vi "mini_test_main_(QMH_ver).vi"() -> ()   [LabVIEW 2015]
doc: "This program is designed to work with CHROMA instruments, models 19052 and 19572, through the SERIAL RS232 or GPIB interfaces; whichever interface is chosen, it must be used in both.\nNOTE: This application was tested with the following interfaces: National Instruments GPIB-USB-HS and HS+, USB-A to RS-232 (DB9) Serial Adapter Cable Tripp Lite U209-000-R, 2 Port Industrial USB to Serial Adapter Hub ICUSB2322I. The one that gave the best result was the Startech interface.\n\nThe application takes configuration parameters from two files: config.ini and VISA_config.ini.\nThe first one configures the test mode and the delay time between the start of the second test and the start of the first one. And the second one configures communication parameters for the chosen interface.\n\nThe application has the ability to test in 4 different modes: The first two modes can perform Hi-Pot and GB testing simultaneously. The second two are single tests, one or the other, Hi-Pot or GB. The four possible modes are described as follows.\n\ntest_mode = 0, performs the sequence Hi-Pot then GB. The tests can be simultaneous or in sequence: Hi-Pot first and then GB. The start of the second one depends on the programmed delay time.\ntest_mode = 1, performs the sequence GB then Hi-Pot. The tests can be simultaneous or in sequence: GB first and then Hi-Pot. The start of the second test depends on the programmed delay time.\ntest_mode = 2, performs the Hi-Pot test only, and is the default test in case no mode is chosen in the config.ini configuration file.\ntest_mode = 3, performs the GB only GB test."
uses:
  controls/UI Data.ctl
  controls/HP Data.ctl
  controls/GB Data.ctl
  controls/Timer Data.ctl
  support/Message Queue/Enqueue Message (Array).vi
  support/Message Queue/Enqueue Message (Single).vi
  <vilib>/Utility/error.llb/Error Cluster From Error Code.vi
  <vilib>/ErrorRing/Error Ring.xnode
  support/Message Queue/Message Queue.lvlib
  support/User Event - Stop/User Event - Stop.lvlib
panel:
  in  "stp tmr":bool caption="stop"
  out "GB Pass/Fail":cluster{"PASS":bool, "FAIL":bool}
  out "HP Pass/Fail":cluster{"PASS":bool, "FAIL":bool}
  out "tst mod":T1(ring) caption="Test mode"
  out "tst time":dbl caption="total test time"
  out "overlap":dbl
  out "2d tst":dbl caption="test time 2"
  out "1st tst":dbl caption="test time 1"
  out "delay":dbl caption="delay time"
  out "GB test":dbl(slide) caption="GB test time [s]" scale=0.0..1.0 scale format="%#_3g"
  out "HP test":dbl(slide) caption="Hi-Pot test time [s]" scale=0.0..1.0 scale format="%#_3g"
  out "I/F type":string caption="Interface type"
  out "GB ID":string="\r\n" caption="GB Instrument ID"
  out "HP ID":string="\r\n" caption="Hi-Pot Instrument ID"
  out "GB tst reslts":string caption="GB test results"
  out "GB tst st":string caption="GB test status"
  out "HP tst rslts":string caption="Hi-Pot test results"
  out "HP tst st":string caption="Hi-Pot test status"
  out "Display":string
  in  "Stop test":bool
  in  "Start test":bool
  in  "Exit Button":bool
  # "QMH version"
  # "Hi-Pot test"
  # "GB test"
  # "Warning. This app is a proof of concept and has no other purpose, \nit is not intended for production. Use at your own risk."
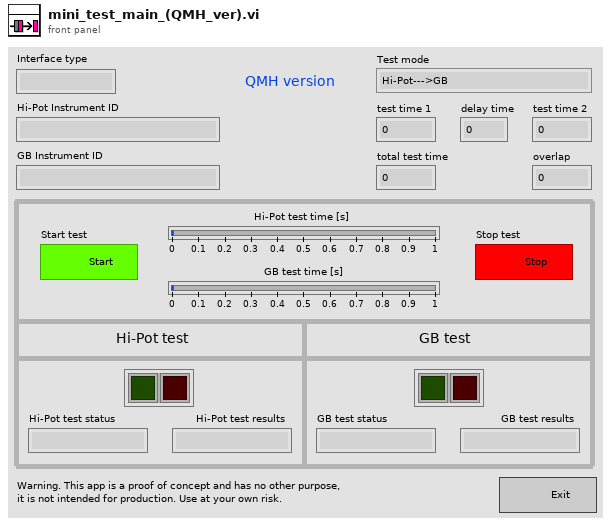
[diagram p1: front panel]
types:
  T1 = enum16{"Hi-Pot--->GB", "GB--->Hi-Pot", "Hi-Pot only", "GB only"}
  T2 = typedef "Timer Data.ctl" = cluster{"Delay time":dbl}
  T3 = typedef "GB Data.ctl" = cluster{"Status GB":string, "Results GB":string, "GB Pass/Fail":cluster{"PASS":bool, "FAIL":bool}}
  T4 = typedef "HP Data.ctl" = cluster{"Status HP":string, "Results HP":string, "HP Pass/Fail":cluster{"PASS":bool, "FAIL":bool}}
  T5 = typedef "UI Data.ctl" = cluster{"Delay Time":dbl, "prms":cluster{"1st tst":dbl, "2nd tst":dbl, "overlap":dbl, "tst time":dbl, "delay":dbl}, "test mode":enum16{"Hi-Pot--->GB", "GB--->Hi-Pot", "Hi-Pot only", "GB only"}, "Start Btn Refnum":refnum<vi>}
  T6 = cluster{"test mode number":string, "test mode":enum16{"Hi-Pot--->GB", "GB--->Hi-Pot", "Hi-Pot only", "GB only"}, "size":i32}
  T7 = cluster{"Rsrc name for 19572":refnum<visa-resource-name>, "Rsrc name for 19052":refnum<visa-resource-name>, "I/F type":string, "VISA2 Inst ID":string, "VISA1 Inst ID":string, "test mode":enum16{"Hi-Pot--->GB", "GB--->Hi-Pot", "Hi-Pot only", "GB only"}}
  T8 = typedef "Message Queue.lvlib/All Message Queues.ctl" = cluster{"Main":refnum<queue>, "GB Test":refnum<queue>, "HP Test":refnum<queue>, "Timer":refnum<queue>}
  T9 = enum8{"Enabled", "Disabled", "Disabled and Grayed Out"}
  T10 = cluster{"1st tst":dbl, "2nd tst":dbl, "overlap":dbl, "tst time":dbl, "delay":dbl}
  T11 = cluster{"1st test":dbl, "2nd test":dbl, "overlap":dbl, "test time":dbl, "delay":dbl}
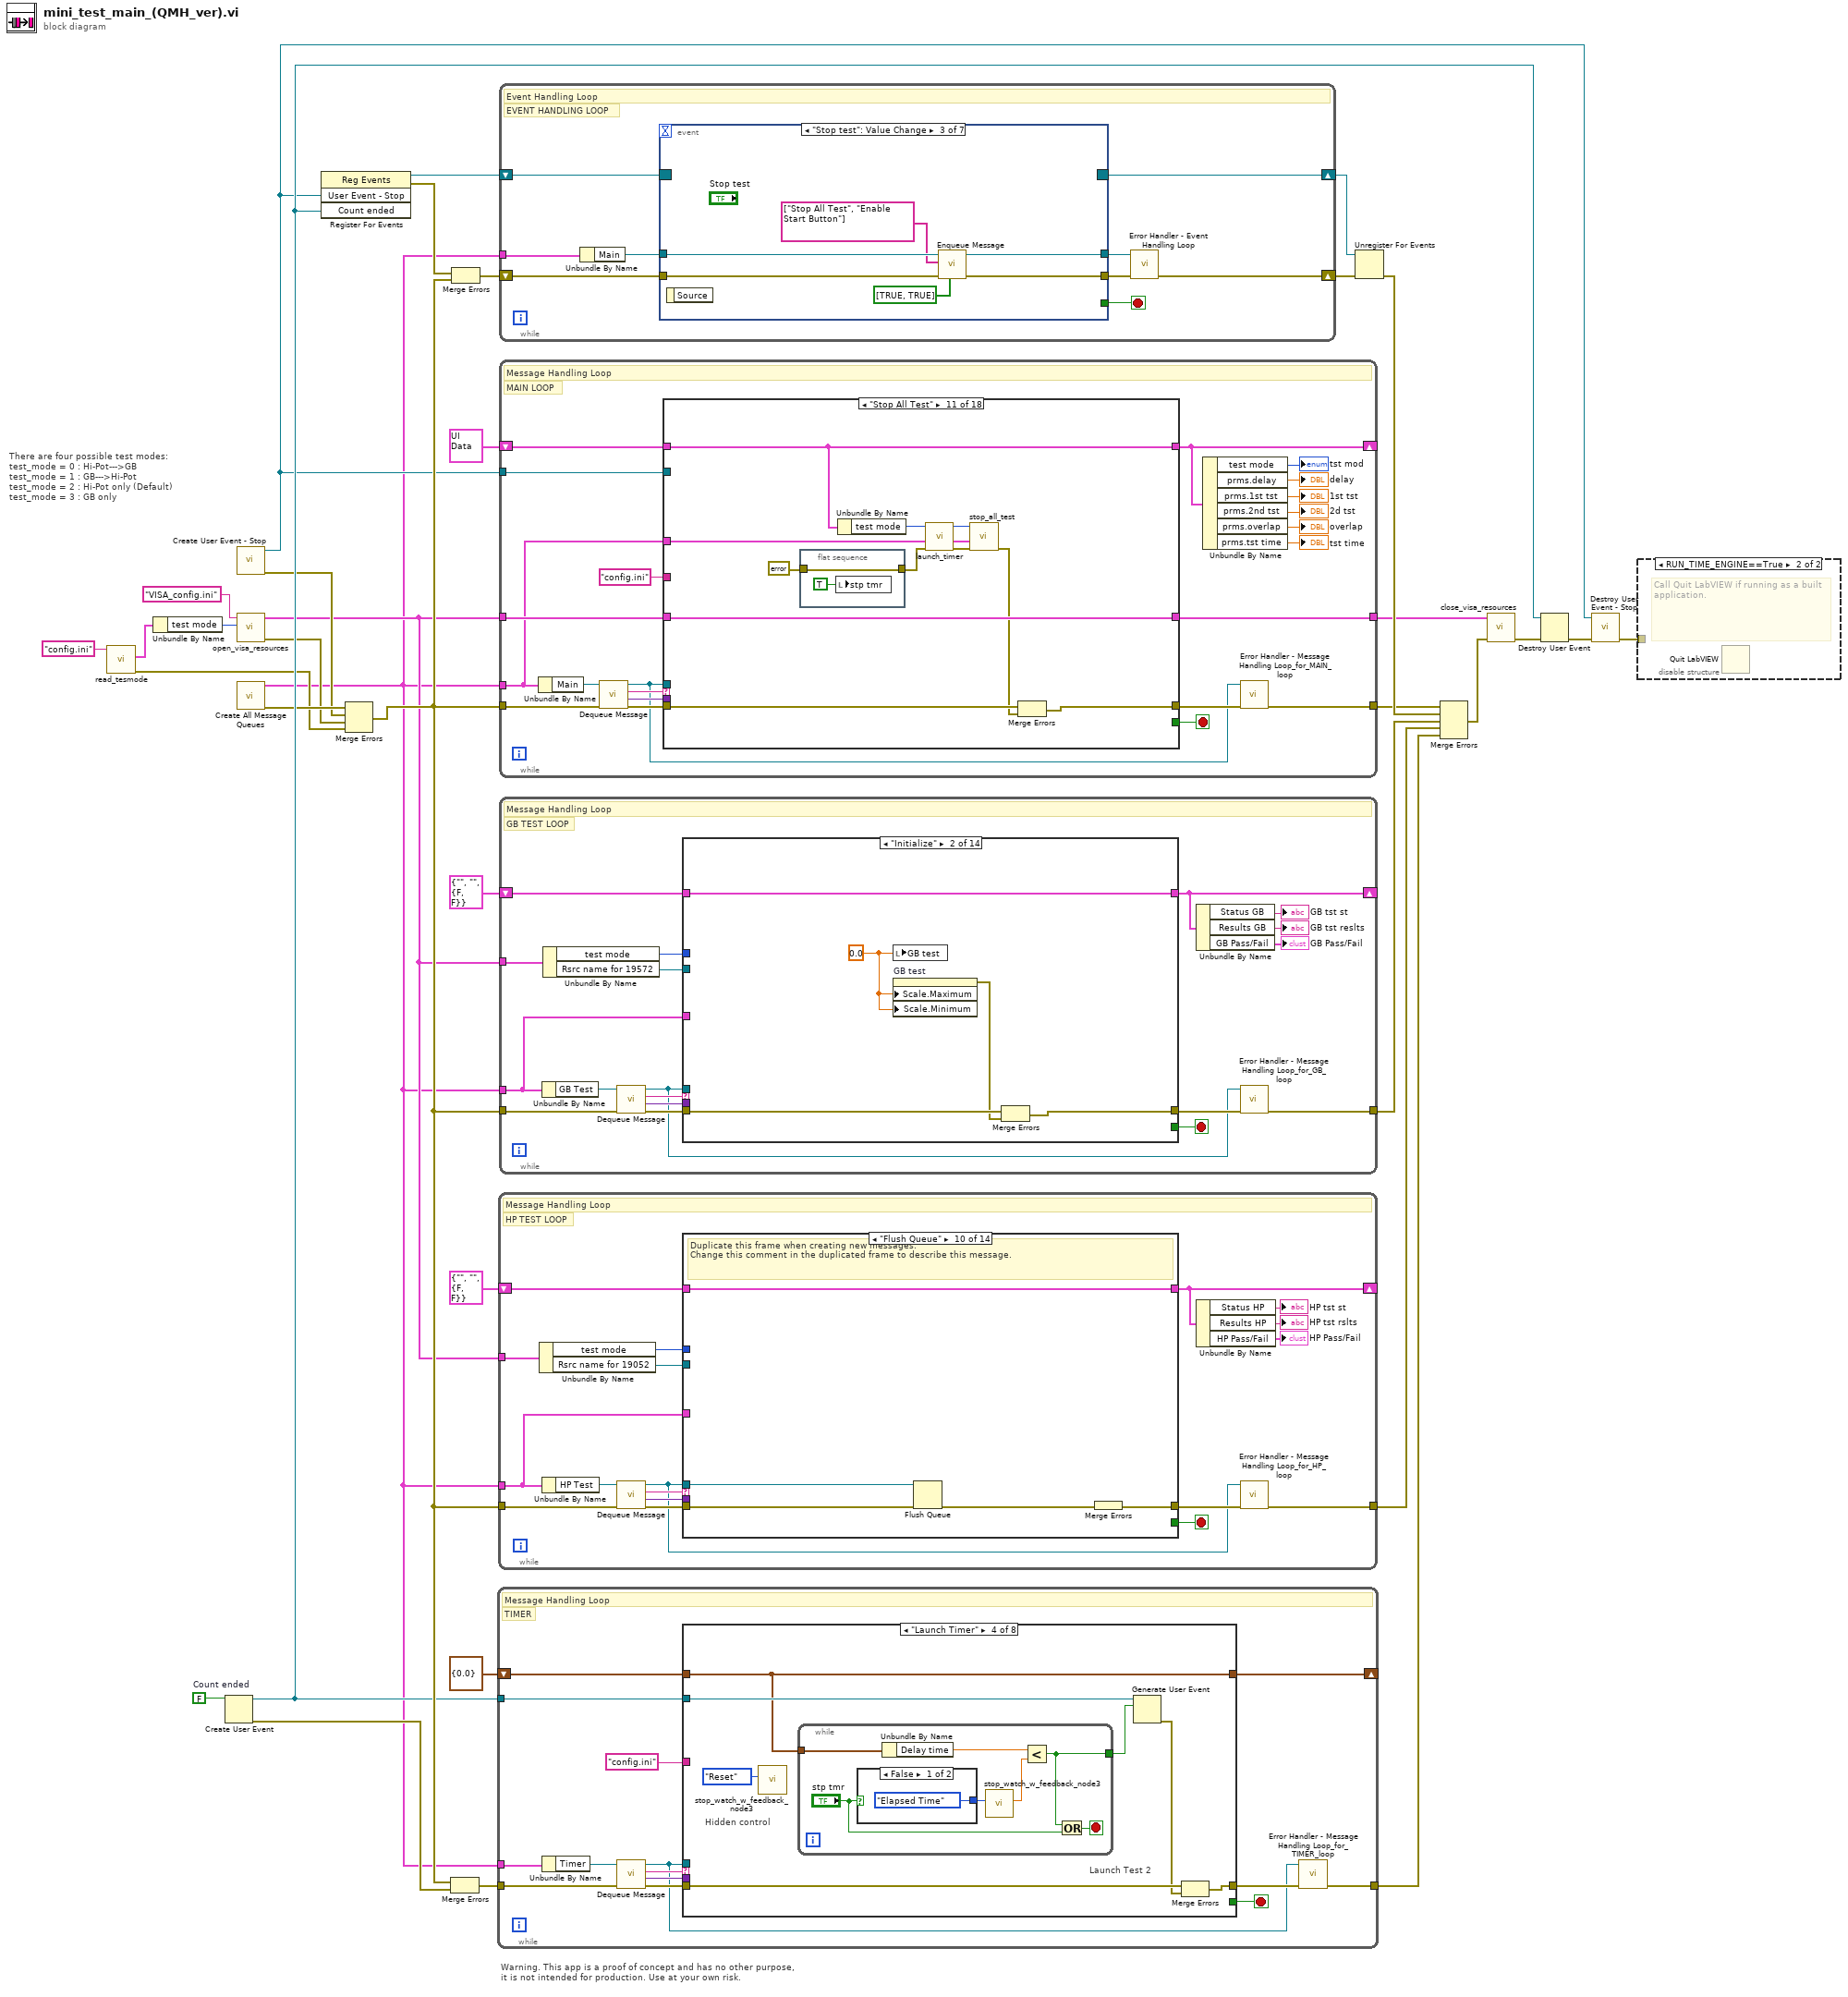
[diagram p0: block diagram]
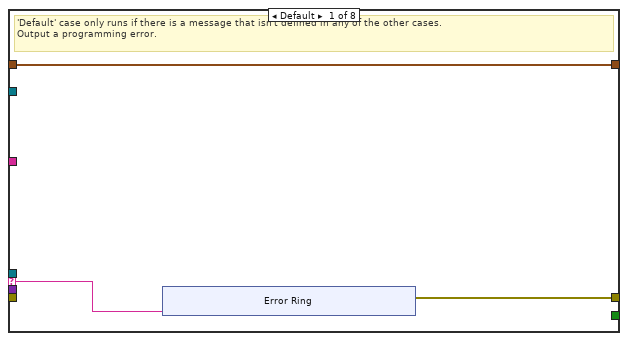
[diagram p2: hidden frame]
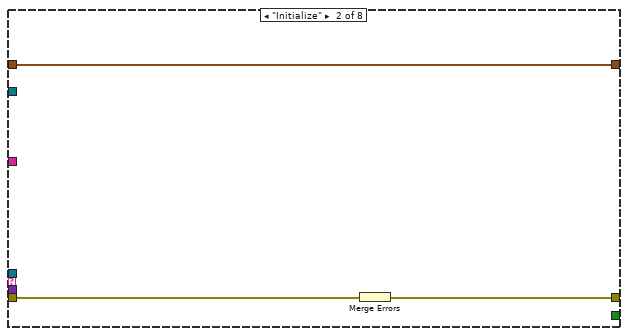
[diagram p3: hidden frame]
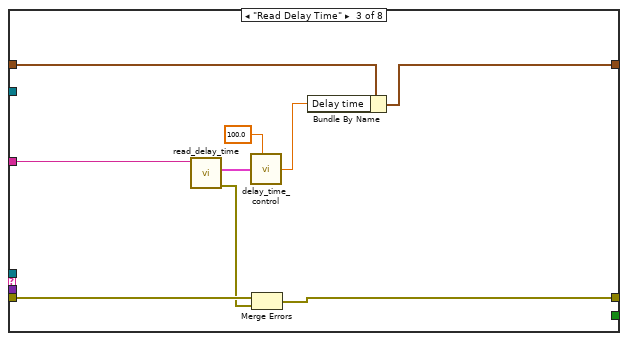
[diagram p4: hidden frame]
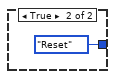
[diagram p5: hidden frame]
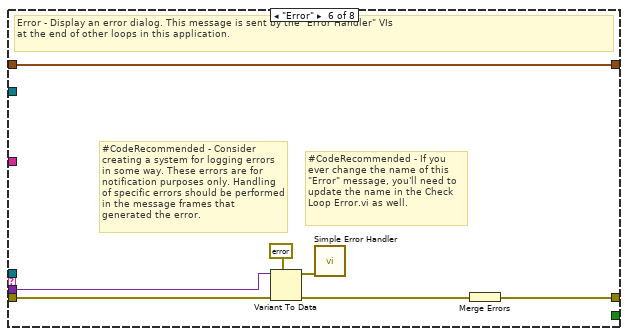
[diagram p7: hidden frame]
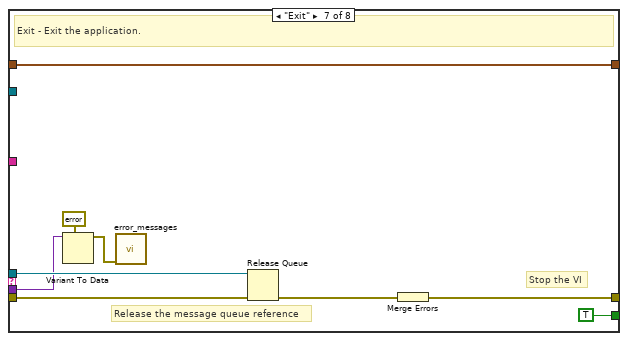
[diagram p8: hidden frame]
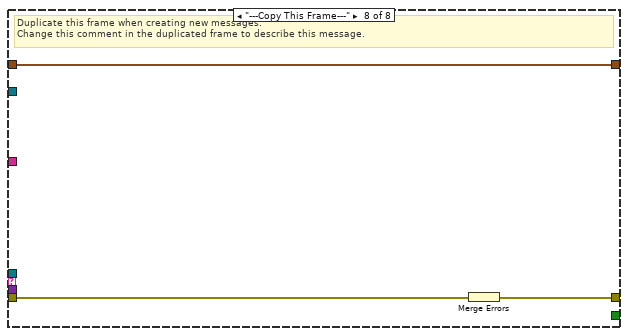
[diagram p9: hidden frame]
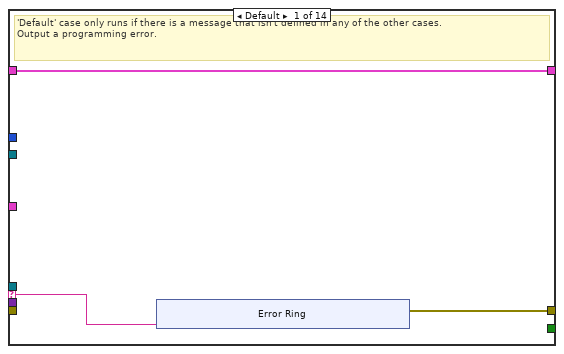
[diagram p10: hidden frame]
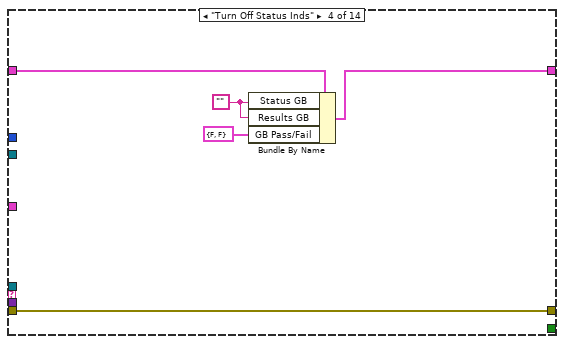
[diagram p12: hidden frame]
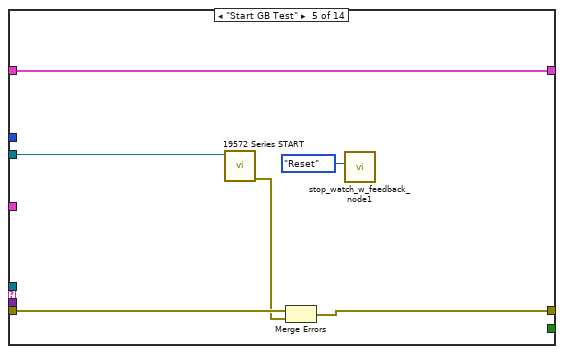
[diagram p13: hidden frame]
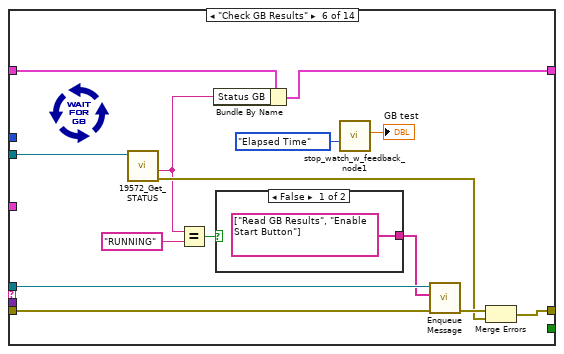
[diagram p14: hidden frame]
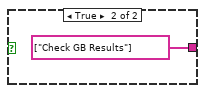
[diagram p15: hidden frame]
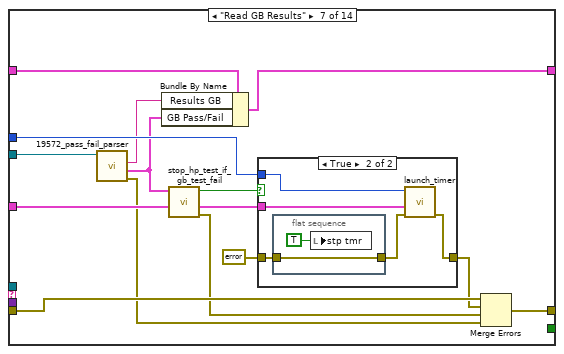
[diagram p16: hidden frame]
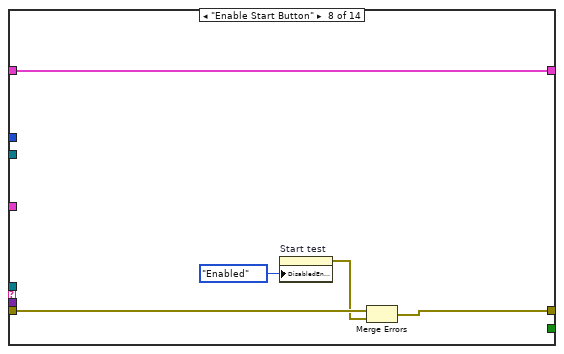
[diagram p18: hidden frame]
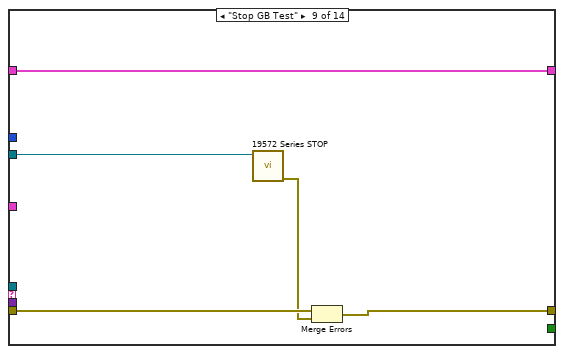
[diagram p19: hidden frame]
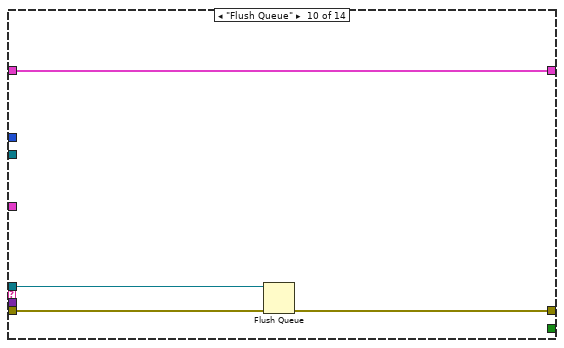
[diagram p20: hidden frame]
diagram:
  w13 = FALSE  # Count ended
  # "Warning. This app is a proof of concept and has no other purpose, \nit is not intended for production. Use at your own risk."
  # "There are four possible test modes:\ntest_mode = 0 : Hi-Pot--->GB\ntest_mode = 1 : GB--->Hi-Pot\ntest_mode = 2 : Hi-Pot only (Default)\ntest_mode = 3 : GB only"
  n1 = call "read_tesmode.vi"("config_file_name"="config.ini") -> ("error out"=w31:errorcluster, "test mode"=w17:T6)  [unwired: 8 in, 1 out]
  n2 = Unbundle By Name(w17) -> ("test mode"=w16:T1)
  n3 = Create User Event(user event datatype=w13) -> (user event=w34:refnum<user-event>, error out=w11:errorcluster)  [unwired: 1 in]
  n4 = call "Create User Event - Stop.vi"() -> ("error out"=w19:errorcluster, "User Event - Stop"=w29:refnum<user-event>)  [unwired: 10 in]
  n5 = call "open_visa_resources.vi"("test mode"=w16, "config file in"="VISA_config.ini") -> ("error out"=w32:errorcluster, "VISA out"=w6:T7)  [unwired: 8 in]
  n6 = call "Create All Message Queues.vi"() -> ("error out"=w33:errorcluster, "Message Queues out"=w5:T8)  [unwired: 10 in]
  n7 = register-events(w29, w34) -> (reference out=w25:refnum<event-registration>, error out=w30:errorcluster)  [unwired: 2 in]
  n8 = Merge Errors(w33, w19, w32, w31) -> (w35:errorcluster)
  n9 = Merge Errors(w35, w11) -> (w12:errorcluster)
  n10 = Merge Errors(w30, w35) -> (w4:errorcluster)
  n11 = while {
    shift-right: [w37] -> _
    shift-left: T2 {"Delay time"=0.0} ("Timer Data") -> [w49]
    tunnel: w12 -> [w48]
    tunnel: [w41] -> w7
    tunnel: w5 -> [w44]
    tunnel: w34 -> [w38]
    stop <- w45 stop-if-true
    # "TIMER"
    # "Message Handling Loop"
    n12 = Unbundle By Name(w44) -> ("Timer"=w43:refnum<queue>)
    n13 = call "Dequeue Message.vi"("error in (no error)"=w48, "Message Queue"=w43) -> ("error out"=w47:errorcluster, "Message Data"=w46:variant, "Message"=w40:string, "dup Message Queue"=w36:refnum<queue>)  [unwired: 6 in]
    n14 = case "Message Cases" shown="\"Launch Timer\"" w40 {
      selector: w40 -> [w50 _ _ _ _ _ _ _]
      tunnel: w36 -> [_ _ _ _ _ _ w105 _]
      tunnel: w47 -> [_ w61 w70 w76 w89 w96 w101 w108]
      tunnel: [w51 w60 w71 w78 w89 w90 w102 w106] -> w42
      tunnel: w49 -> [w52 w62 w69 w73 w88 w95 w97 w107]
      tunnel: [w52 w62 w65 w73 w88 w95 w97 w107] -> w37
      tunnel: [_ _ _ _ _ _ TRUE _] -> w45
      tunnel: w46 -> [_ _ _ _ _ w94 w99 _]
      tunnel: "config.ini" -> [_ _ w67 _ _ _ _ _]
      tunnel: w38 -> [_ _ _ w77 _ _ _ _]
      frame Default {
        # "'Default' case only runs if there is a message that isn't defined in any of the other cases. \nOutput a programming error."
        n15 = xnode "Error Ring"("parameter 0"=w50) -> ("error out"=w51:errorcluster)
      }
      frame "Initialize" {
        n16 = Merge Errors(w61) -> (w60:errorcluster)
      }
      frame "Read Delay Time" {
        n17 = call "read_delay_time.vi"("config_file_name"=w67) -> ("error out"=w64:errorcluster, "values"=w68:cluster{"delay_time":string})  [unwired: 8 in, 1 out]
        n18 = call "delay_time_control.vi"("Higher limit"=100.0, "values in"=w68) -> ("delay time"=w63:dbl)  [unwired: 5 in]
        n19 = Merge Errors(w70, w64) -> (w71:errorcluster)
        n20 = Bundle By Name(cluster=w69, "Delay time"=w63) -> (w65:T2)
      }
      frame "Launch Timer" {
        # "Launch Test 2"
        # "Hidden control"
        n21 = call "stop_watch_w_feedback_node3.vi"("Command"=enum16{"Elapsed Time", "Reset"}."Reset") -> ()  [unwired: 10 in, 1 out]
        n22 = while {
          tunnel: w73 -> [w85]
          tunnel: [w80] -> w72
          stop <- w84 stop-if-true
          n23 = case shown="False" "stp tmr" {
            tunnel: [enum16{"Elapsed Time", "Reset"}."Elapsed Time" ("Command") enum16{"Elapsed Time", "Reset"}."Reset" ("Command")] -> w83
            frame False {
            }
            frame True {
            }
          }
          n24 = Unbundle By Name(w85) -> ("Delay time"=w81:dbl)
          n25 = call "stop_watch_w_feedback_node3.vi"("Command"=w83) -> ("Elapsed Time"=w82:dbl)  [unwired: 10 in]
          n26 = Less?(x=w81, y=w82) -> (x < y?=w80:bool)
          n27 = Or(x=w80, y="stp tmr") -> (x .or. y?=w84:bool)
        }
        n28 = Generate User Event(user event=w77, event data cluster=w72) -> (error out=w75:errorcluster)  [unwired: 2 in, 1 out]
        n29 = Merge Errors(w76, w75) -> (w78:errorcluster)
      }
      frame "Idle" {
      }
      frame "Error" {
        # "#CodeRecommended - If you ever change the name of this \"Error\" message, you'll need to update the name in the Check Loop Error.vi as well."
        # "#CodeRecommended - Consider creating a system for logging errors in some way. These errors are for notification purposes only. Handling of specific errors should be performed in the message frames that generated the error."
        # "Error - Display an error dialog. This message is sent by the \"Error Handler\" VIs \nat the end of other loops in this application."
        n30 = Variant To Data(error in=w96, type=errorcluster {"status"=FALSE, "code"=0, "source"=""} ("error constant"), Variant=w94) -> (data=w92:errorcluster, error out=w91:errorcluster)
        n31 = call <vilib>:"Simple Error Handler.vi"("error in (no error)"=w92) -> ()  [unwired: 4 in, 5 out]
        n32 = Merge Errors(w91) -> (w90:errorcluster)
      }
      frame "Exit" {
        # "Stop the VI"
        # "Release the message queue reference"
        # "Exit - Exit the application."
        n33 = Variant To Data(type=errorcluster {"status"=FALSE, "code"=0, "source"=""} ("error constant"), Variant=w99) -> (data=w98:errorcluster)  [unwired: 1 in, 1 out]
        n34 = call "error_messages.vi"("error in (no error)"=w98) -> ()  [unwired: 10 in, 1 out]
        n35 = Release Queue(queue=w105, error in (no error)=w101) -> (error out=w103:errorcluster)  [unwired: 1 in, 2 out]
        n36 = Merge Errors(w103) -> (w102:errorcluster)
      }
      frame "---Copy This Frame---" {
        # "Duplicate this frame when creating new messages.\nChange this comment in the duplicated frame to describe this message."
        n37 = Merge Errors(w108) -> (w106:errorcluster)
      }
    }
    n38 = call "Error Handler - Message Handling Loop_for_TIMER_loop.vi"("error in (no error)"=w42, "Message Queue"=w36) -> ("dup error in"=w41:errorcluster)  [unwired: 8 in, 1 out]
  }
  n39 = while {
    shift-right: [w119] -> _
    shift-left: T4 {"Status HP"="", "Results HP"="", "HP Pass/Fail"={"PASS"=FALSE, "FAIL"=FALSE}} ("HP Data") -> [w126]
    tunnel: w35 -> [w125]
    tunnel: [w114] -> w24
    tunnel: w6 -> [w121]
    tunnel: w5 -> [w111]
    stop <- w122 stop-if-true
    # "HP TEST LOOP"
    # "Message Handling Loop"
    n40 = Unbundle By Name(w121) -> ("test mode"=w110:T1, "Rsrc name for 19052"=w120:refnum<visa-resource-name>)
    n41 = Unbundle By Name(w111) -> ("HP Test"=w116:refnum<queue>)
    n42 = call "Dequeue Message.vi"("error in (no error)"=w125, "Message Queue"=w116) -> ("error out"=w124:errorcluster, "Message Data"=w123:variant, "Message"=w113:string, "dup Message Queue"=w109:refnum<queue>)  [unwired: 6 in]
    n43 = case "Message Cases" shown="\"Flush Queue\"" w113 {
      selector: w113 -> [w127 _ _ _ _ _ _ _ _ _ _ _ _ _]
      tunnel: w109 -> [_ _ _ _ _ w165 _ _ _ w206 _ _ w235 _]
      tunnel: w124 -> [_ w139 w143 w148 w153 w167 w185 w198 w200 w205 w212 w221 w231 w238]
      tunnel: [w128 w138 w143 w148 w152 w168 w184 w195 w202 w207 w213 w215 w232 w236] -> w115
      tunnel: w126 -> [w129 w141 w142 w145 w149 w163 w182 w197 w203 w208 w214 w220 w226 w237]
      tunnel: [w129 w141 w142 w144 w149 w162 w181 w197 w203 w208 w214 w220 w225 w237] -> w119
      tunnel: [_ _ _ _ _ _ _ _ _ _ _ _ TRUE _] -> w122
      tunnel: w123 -> [_ _ _ _ _ _ _ _ _ _ w211 w219 w229 _]
      tunnel: w120 -> [_ _ _ _ w154 w164 w183 _ w201 _ _ _ _ _]
      tunnel: w111 -> [_ _ _ _ _ _ w178 _ _ _ _ _ _ _]
      tunnel: w110 -> [_ _ _ _ _ _ w176 _ _ _ _ _ _ _]
      frame Default {
        # "'Default' case only runs if there is a message that isn't defined in any of the other cases. \nOutput a programming error."
        n44 = xnode "Error Ring"("parameter 0"=w127) -> ("error out"=w128:errorcluster)
      }
      frame "Initialize" {
        w140 = 0.0
        n45 = local write "HP test"(w140) -> ()
        n46 = property on="HP test" class="Slide (strict)"("Scale.Maximum"=w140, "Scale.Minimum"=w140) -> (error out=w137:errorcluster)  [unwired: 2 in, 1 out]
        n47 = Merge Errors(w139, w137) -> (w138:errorcluster)
      }
      frame "Idle" {
      }
      frame "Turn Off Status Inds" {
        w146 = ""
        n48 = Bundle By Name(cluster=w145, "Status HP"=w146, "Results HP"=w146, "HP Pass/Fail"=cluster{"PASS":bool, "FAIL":bool} {"PASS"=FALSE, "FAIL"=FALSE} ("GB Pass/Fail")) -> (w144:T4)
      }
      frame "Start HP Test" {
        n49 = call "19052 Series START.vi"("VISA resource in"=w154) -> ("error out"=w151:errorcluster)  [unwired: 9 in, 1 out]
        n50 = Merge Errors(w153, w151) -> (w152:errorcluster)
        n51 = call "stop_watch_w_feedback_node2.vi"("Command"=enum16{"Elapsed Time", "Reset"}."Reset") -> ()  [unwired: 10 in, 1 out]
      }
      frame "Check HP Results" {
        n52 = call "19052_Get_STATUS.vi"("VISA resource in"=w164) -> ("error out"=w158:errorcluster, "Status"=w157:string)  [unwired: 8 in, 1 out]
        n53 = Equal?(x=w157, y="RUNNING") -> (x = y?=w160:bool)
        n54 = Bundle By Name(cluster=w163, "Status HP"=w157) -> (w162:T4)
        n55 = case shown="False" w160 {
          tunnel: [string[] ["Read HP Results", "Enable Start Button"] string[] ["Check HP Results"]] -> w159
          frame False {
          }
          frame True {
          }
        }
        n56 = call "stop_watch_w_feedback_node2.vi"("Command"=enum16{"Elapsed Time", "Reset"}."Elapsed Time") -> ("Elapsed Time"=→"HP test":dbl)  [unwired: 10 in]
        n57 = call-poly "Enqueue Message.vi"("error in (no error)"=w167, "Message Array"=w159, "Message Queue"=w165) -> ("error out"=w166:errorcluster)  [unwired: 7 in, 1 out]
        n58 = Merge Errors(w166, w158) -> (w168:errorcluster)
      }
      frame "Read HP Results" {
        n59 = call "19052_pass_fail_parser.vi"("VISA resource in"=w183) -> ("error out"=w177:errorcluster, "Pass/Fail"=w179:cluster{"PASS":bool, "FAIL":bool}, "Code Results"=w180:string)  [unwired: 7 in, 1 out]
        n60 = Bundle By Name(cluster=w182, "Results HP"=w180, "HP Pass/Fail"=w179) -> (w181:T4)
        n61 = call "stop_gb_test_if_hp_test_fail.vi"("Message Queues in"=w178, "Pass/Fail"=w179) -> ("error out"=w171:errorcluster, "Message Queues out"=w174:T8, "Fail?"=w173:bool)  [unwired: 7 in]
        n62 = case shown="True" w173 {
          tunnel: [w186 w190] -> w172
          tunnel: errorcluster {"status"=FALSE, "code"=0, "source"=""} ("error constant") -> [w186 w189]
          tunnel: w176 -> [_ w188]
          tunnel: w174 -> [_ w187]
          frame False {
          }
          frame True {
            n63 = flat-sequence {
              tunnel: w189 -> [w192]
              tunnel: [w192] -> w191
              frame #0 {
                n64 = local write "stp tmr"(TRUE ("stp tmr")) -> ()
              }
            }
            n65 = call "launch_timer.vi"("error in (no error)"=w191, "Message Queues in"=w187, "test mode in"=w188) -> ("error out"=w190:errorcluster)  [unwired: 6 in, 2 out]
          }
        }
        n66 = Merge Errors(w185, w177, w172, w171) -> (w184:errorcluster)
      }
      frame "Enable Start Button" {
        n67 = property on="Start test" class="Bool"("DisabledEnum"=T9."Enabled" ("Disabled")) -> (error out=w194:errorcluster)  [unwired: 2 in, 1 out]
        n68 = Merge Errors(w198, w194) -> (w195:errorcluster)
      }
      frame "Stop HP Test" {
        n69 = call "19052 Series STOP.vi"("VISA resource in"=w201) -> ("error out"=w199:errorcluster)  [unwired: 9 in, 1 out]
        n70 = Merge Errors(w200, w199) -> (w202:errorcluster)
      }
      frame "Flush Queue" {
        # "Duplicate this frame when creating new messages.\nChange this comment in the duplicated frame to describe this message."
        n71 = Flush Queue(queue=w206, error in (no error)=w205) -> (error out=w204:errorcluster)  [unwired: 2 out]
        n72 = Merge Errors(w204) -> (w207:errorcluster)
      }
      frame "Update HP Display" {
        # "#CodeRecommended - If you wish to decouple the Message Handling Loop from your user interface, consider creating User Events (like the \"Stop\" event in this VI) to message the Event Handling Loop whenever the user interface needs updating."
        # "Update Display - Convert the message data to a string to display in the Data Display indicator."
        n73 = Variant To Data(error in=w212, type="", Variant=w211) -> (error out=w209:errorcluster)  [unwired: 1 out]
        n74 = Merge Errors(w209) -> (w213:errorcluster)
      }
      frame "Error" {
        # "#CodeRecommended - If you ever change the name of this \"Error\" message, you'll need to update the name in the Check Loop Error.vi as well."
        # "#CodeRecommended - Consider creating a system for logging errors in some way. These errors are for notification purposes only. Handling of specific errors should be performed in the message frames that generated the error."
        # "Error - Display an error dialog. This message is sent by the \"Error Handler\" VIs \nat the end of other loops in this application."
        n75 = Variant To Data(error in=w221, type=errorcluster {"status"=FALSE, "code"=0, "source"=""} ("error constant"), Variant=w219) -> (data=w217:errorcluster, error out=w216:errorcluster)
        n76 = call <vilib>:"Simple Error Handler.vi"("error in (no error)"=w217) -> ()  [unwired: 4 in, 5 out]
        n77 = Merge Errors(w216) -> (w215:errorcluster)
      }
      frame "Exit" {
        w224 = ""
        w228 = 0.0 ("HP test")
        # "Stop the VI"
        # "Release the message queue reference"
        # "#CodeNeeded - Add any required cleanup code here. Note that if 'Exit' was called as a result of an error, an error dialog will be displayed. Add any custom error handling for an 'Exit' condition here as well."
        # "Exit - Exit the application."
        n78 = Variant To Data(type=errorcluster {"status"=FALSE, "code"=0, "source"=""} ("error constant"), Variant=w229) -> (data=w223:errorcluster)  [unwired: 1 in, 1 out]
        n79 = call "error_messages.vi"("error in (no error)"=w223) -> ()  [unwired: 10 in, 1 out]
        n80 = Release Queue(queue=w235, error in (no error)=w231) -> (error out=w233:errorcluster)  [unwired: 1 in, 2 out]
        n81 = property on="HP test" class="Slide (strict)"("Scale.Maximum"=w228, "Scale.Minimum"=w228) -> (error out=w227:errorcluster)  [unwired: 2 in, 1 out]
        n82 = local write "HP test"(w228) -> ()
        n83 = Merge Errors(w233, w227) -> (w232:errorcluster)
        n84 = Bundle By Name(cluster=w226, "Status HP"=w224, "Results HP"=w224, "HP Pass/Fail"=cluster{"PASS":bool, "FAIL":bool} {"PASS"=FALSE, "FAIL"=FALSE}) -> (w225:T4)
      }
      frame "---Copy This Frame---" {
        # "Duplicate this frame when creating new messages.\nChange this comment in the duplicated frame to describe this message."
        n85 = Merge Errors(w238) -> (w236:errorcluster)
      }
    }
    n86 = Unbundle By Name(w119) -> ("Status HP"=→"HP tst st":string, "Results HP"=→"HP tst rslts":string, "HP Pass/Fail"=→"HP Pass/Fail":cluster{"PASS":bool, "FAIL":bool})
    n87 = call "Error Handler - Message Handling Loop_for_HP_loop.vi"("error in (no error)"=w115, "Message Queue"=w109) -> ("dup error in"=w114:errorcluster)  [unwired: 8 in, 1 out]
  }
  n88 = while {
    shift-right: [w246] -> w27
    shift-left: w25 -> [w247]
    tunnel: w5 -> [w242]
    shift-right: [w239] -> w26
    shift-left: w4 -> [w240]
    stop <- w244 stop-if-true
    # "EVENT HANDLING LOOP"
    # "Event Handling Loop"
    n89 = Unbundle By Name(w242) -> ("Main"=w241:refnum<queue>)
    n90 = event shown="[2] \"Stop test\": Value Change" {
      selector: w247 -> [_ _ _ _ _ _ _]
      dyn-events: [_ _ _ _ _ _ _] -> w246
      timeout: _ -> [_ _ _ _ _ _ _]
      tunnel: [_ _ _ _ _ _ TRUE ("Discard?")] -> w244
      tunnel: w241 -> [w253 w258 w271 w278 w281 w287 w291]
      tunnel: [w249 w255 w268 w277 w280 w284 w288] -> w245
      tunnel: [w252 w257 w270 w276 w281 w286 w291] -> w243
      tunnel: w240 -> [w251 w256 w269 w275 w280 w285 w288]
      event "Start test": Value Change {
        n91 = event-data() -> ()  [unwired: 1 in, 1 out]
        n92 = call-poly "Enqueue Message.vi"("error in (no error)"=w251, "Message Array"=string[] ["Launch Test 1", "Idle"], "Message Queue"=w253) -> ("error out"=w250:errorcluster, "dup Message Queue"=w252:refnum<queue>)  [unwired: 7 in]
        n93 = Merge Errors(w250) -> (w249:errorcluster)
      }
      event User Event {
        n94 = event-data() -> ("Count ended"=w254:bool)  [unwired: 1 in]
        n95 = case shown="True" w254 {
          tunnel: w258 -> [w260 w265]
          tunnel: [w260 w264] -> w257
          tunnel: w256 -> [w259 w263]
          tunnel: [w259 w262] -> w255
          frame False {
          }
          frame True {
            n96 = call-poly "Enqueue Message.vi"("error in (no error)"=w263, "Message Array"=string[] ["Launch Test 2", "Idle"], "Message Queue"=w265) -> ("error out"=w262:errorcluster, "dup Message Queue"=w264:refnum<queue>)  [unwired: 7 in]
          }
        }
      }
      event "Stop test": Value Change {
        n97 = event-data() -> ()  [unwired: 1 in, 1 out]
        n98 = call-poly "Enqueue Message.vi"("Priority Message? Array"=bool[] [TRUE, TRUE], "error in (no error)"=w269, "Message Array"=string[] ["Stop All Test", "Enable Start Button"], "Message Queue"=w271) -> ("error out"=w268:errorcluster, "dup Message Queue"=w270:refnum<queue>)  [unwired: 6 in]
      }
      event Panel Close? {
        # "Send the 'Confirm Quit' message if the user closes the panel of the VI. Discard the event so the 'Confirm Quit' message has a chance to run."
        n99 = event-data() -> ()  [unwired: 1 in, 1 out]
        n100 = call-poly "Enqueue Message.vi"("Priority Message? (F)"=TRUE, "error in (no error)"=w275, "Message Data"="Are you sure?", "Message"="Confirm Quit", "Message Queue"=w278) -> ("error out"=w277:errorcluster, "dup Message Queue"=w276:refnum<queue>)  [unwired: 5 in]
        n101 = event-data("Discard?"=TRUE) -> ()  [unwired: 1 in, 1 out]
      }
      event Application Instance Close {
        # "#CodeRecommended - When a project closes, all VIs within that project are aborted and leave memory. However, any code placed in this event frame is guaranteed to run to completion, so add any cleanup code that absolutely must happen here."
        n102 = event-data() -> ()  [unwired: 1 in, 1 out]
      }
      event "Exit Button": Value Change {
        n103 = event-data() -> ()  [unwired: 1 in, 1 out]
        n104 = call-poly "Enqueue Message.vi"("Priority Message? Array"=bool[] [TRUE, TRUE, TRUE], "error in (no error)"=w285, "Message Array"=string[] ["Turn Off Indicators", "Exit", "Enable Start Button"], "Message Queue"=w287) -> ("error out"=w284:errorcluster, "dup Message Queue"=w286:refnum<queue>)  [unwired: 6 in]
      }
      event User Event {
        # "The Message Handling Loop processed an \"Exit\" message, which fired this event to stop the Event Handling Loop."
        n105 = event-data() -> ()  [unwired: 1 in, 1 out]
        n106 = local write "Display"("\"Exit\" button pressed" ("VI Stopped")) -> ()
      }
    }
    n107 = call "Error Handler - Event Handling Loop.vi"("error in (no error)"=w245, "Message Queue"=w243) -> ("dup error in"=w239:errorcluster)  [unwired: 8 in, 1 out]
  }
  n108 = while {
    shift-right: [w301] -> _
    shift-left: T5 {"Delay Time"=0.0, "prms"={"1st tst"=0.0, "2nd tst"=0.0, "overlap"=0.0, "tst time"=0.0, "delay"=0.0}, "test mode"=enum."Hi-Pot--->GB", "Start Btn Refnum"=refnum} ("UI Data") -> [w312]
    tunnel: w29 -> [w311]
    tunnel: w35 -> [w310]
    tunnel: [w307] -> w23
    tunnel: w5 -> [w295]
    tunnel: w6 -> [w303]
    tunnel: [w302] -> w22
    stop <- w306 stop-if-true
    # "MAIN LOOP"
    # "Message Handling Loop"
    n109 = Unbundle By Name(w295) -> ("Main"=w304:refnum<queue>)
    n110 = call "Dequeue Message.vi"("error in (no error)"=w310, "Message Queue"=w304) -> ("error out"=w309:errorcluster, "Message Data"=w308:variant, "Message"=w305:string, "dup Message Queue"=w292:refnum<queue>)  [unwired: 6 in]
    n111 = case "Message Cases" shown="\"Stop All Test\"" w305 {
      selector: w305 -> [w315 _ _ _ _ _ _ _ _ _ _ _ _ _ _ _ _ _]
      tunnel: w292 -> [_ _ _ _ _ _ _ _ w400 w411 _ _ _ _ w464 _ w491 _]
      tunnel: w309 -> [_ w333 w342 w352 w363 w375 w378 w387 w403 w416 w429 w438 w444 w454 w468 w477 w487 w496]
      tunnel: [w316 w334 w341 w351 w362 w366 w378 w386 w405 w417 w428 w436 w445 w449 w466 w477 w489 w494] -> w313
      tunnel: w312 -> [w317 w326 w340 w344 w355 w367 w377 w382 w394 w413 w421 w435 w446 w453 w467 w474 w479 w495]
      tunnel: [w317 w325 w339 w343 w356 w367 w377 w382 w394 w413 w421 w435 w446 w453 w467 w473 w479 w495] -> w301
      tunnel: [_ _ _ _ _ _ _ _ _ _ _ _ _ _ _ _ TRUE _] -> w306
      tunnel: w308 -> [_ _ _ _ _ _ _ _ _ _ _ _ w443 w452 w459 _ w485 _]
      tunnel: w311 -> [_ _ _ _ _ _ _ _ _ _ _ _ _ _ _ _ w488 _]
      tunnel: w303 -> [w314 w335 w338 w350 w354 w374 w376 w385 w404 w414 w427 w437 w439 w448 w463 w476 w492 w493]
      tunnel: [w314 w335 w338 w350 w354 w374 w376 w385 w404 w414 w427 w437 w439 w448 w463 w476 w492 w493] -> w302
      tunnel: w295 -> [_ _ _ _ _ _ _ _ w396 w408 w426 _ _ _ _ _ w480 _]
      tunnel: "config.ini" -> [_ _ _ w346 _ _ _ _ _ _ _ _ _ _ _ _ _ _]
      frame Default {
        # "'Default' case only runs if there is a message that isn't defined in any of the other cases. \nOutput a programming error."
        n112 = xnode "Error Ring"("parameter 0"=w315) -> ("error out"=w316:errorcluster)
      }
      frame "Initialize" {
        # "Bundle control references and a sample string value."
        # "Initialize - All initialization work should take place in this message, since other loops can potentially enqueue messages that execute immediately after this one."
        n113 = control-ref of="Start test"() -> (w327:refnum<vi>)
        n114 = invoke on="Exit Button" class="Bool" method="Reinit To Default"() -> (error out=w331:errorcluster)  [unwired: 3 in, 2 out]
        n115 = invoke on="Stop test" class="Bool" method="Reinit To Default"() -> (error out=w332:errorcluster)  [unwired: 3 in, 2 out]
        n116 = Unbundle By Name(w335) -> ("VISA1 Inst ID"=→"GB ID":string, "VISA2 Inst ID"=→"HP ID":string, "I/F type"=→"I/F type":string)
        n117 = Bundle By Name(cluster=w326, "Start Btn Refnum"=w327) -> (w325:T5)
        n118 = invoke on="Start test" class="Bool" method="Reinit To Default"(error in=w332) -> (error out=w330:errorcluster)  [unwired: 2 in, 2 out]
        n119 = Merge Errors(w333, w331, w330) -> (w334:errorcluster)
      }
      frame "Get Test Mode" {
        # "Duplicate this frame when creating new messages.\nChange this comment in the duplicated frame to describe this message."
        n120 = Unbundle By Name(w338) -> ("test mode"=w337:T1)
        n121 = Merge Errors(w342) -> (w341:errorcluster)
        n122 = Bundle By Name(cluster=w340, "test mode"=w337) -> (w339:T5)
      }
      frame "Read Delay Time" {
        # "Duplicate this frame when creating new messages.\nChange this comment in the duplicated frame to describe this message."
        n123 = call "read_delay_time.vi"("config_file_name"=w346) -> ("error out"=w345:errorcluster, "values"=w349:cluster{"delay_time":string})  [unwired: 8 in, 1 out]
        n124 = Merge Errors(w352, w345) -> (w351:errorcluster)
        n125 = call "delay_time_control.vi"("Higher limit"=100.0, "values in"=w349) -> ("delay time"=w347:dbl)  [unwired: 5 in]
        n126 = Bundle By Name(cluster=w344, "Delay Time"=w347) -> (w343:T5)
      }
      frame "Read Test Params" {
        # "Duplicate this frame when creating new messages.\nChange this comment in the duplicated frame to describe this message."
        n127 = Unbundle By Name(w355) -> ("Delay Time"=w358:dbl, "test mode"=w357:T1)
        n128 = Unbundle By Name(w354) -> ("Rsrc name for 19052"=w359:refnum<visa-resource-name>, "Rsrc name for 19572"=w360:refnum<visa-resource-name>)
        n129 = call "test_definitions_module.vi"("Delay time"=w358, "VISA resource in 19572"=w360, "VISA resource in 19052"=w359, "test mode"=w357) -> ("error out"=w353:errorcluster, "Mode parameters"=w361:T11)  [unwired: 6 in]
        n130 = Bundle By Name(cluster=w355, "prms"=w361) -> (w356:T5)
        n131 = Merge Errors(w363, w353) -> (w362:errorcluster)
      }
      frame "Set Slides" {
        w373 = 0.0
        n132 = Unbundle By Name(w367) -> ("prms.1st tst"=w369:dbl, "prms.2nd tst"=w370:dbl, "test mode"=w368:T1)
        n133 = call "test_number_selector.vi"("1st tst in"=w369, "2nd tst in"=w370, "test mode"=w368) -> ("1st tst out"=w372:dbl, "2nd tst out"=w371:dbl)  [unwired: 2 in]
        n134 = property on="HP test" class="Slide (strict)"("Scale.Maximum"=w372, "Scale.Minimum"=w373) -> (error out=w364:errorcluster)  [unwired: 2 in, 1 out]
        n135 = property on="GB test" class="Slide (strict)"("Scale.Maximum"=w371, "Scale.Minimum"=w373) -> (error out=w365:errorcluster)  [unwired: 2 in, 1 out]
        n136 = Merge Errors(w375, w364, w365) -> (w366:errorcluster)
      }
      frame "Idle" {
      }
      frame "Disable Start Button" {
        # "Duplicate this frame when creating new messages.\nChange this comment in the duplicated frame to describe this message."
        n137 = Unbundle By Name(w382) -> ("Start Btn Refnum"=w381:refnum<vi>)
        n138 = invoke on="GB test" class="Slide (strict)" method="Reinit To Default"() -> (error out=w383:errorcluster)  [unwired: 3 in, 2 out]
        n139 = invoke on="HP test" class="Slide (strict)" method="Reinit To Default"() -> (error out=w384:errorcluster)  [unwired: 3 in, 2 out]
        n140 = property class="Bool"(reference=w381, "DisabledEnum"=T9."Disabled and Grayed Out" ("Disabled")) -> (error out=w379:errorcluster)  [unwired: 1 in, 1 out]
        n141 = Merge Errors(w387, w379, w383, w384) -> (w386:errorcluster)
      }
      frame "Launch Test 1" {
        # "Something - Replace this message with functionality for your own application."
        n142 = Unbundle By Name(w394) -> ("test mode"=w395:T1)
        n143 = call "stop_all_test.vi"("Message Queues in"=w396, "test mode in"=w395) -> ("error out"=w397:errorcluster, "Message Queues out"=w393:T8, "test mode out"=w388:T1)  [unwired: 7 in]
        n144 = flat-sequence {
          tunnel: w397 -> [w406]
          tunnel: [w406] -> w398
          frame #0 {
            n145 = local write "stp tmr"(FALSE ("stp tmr")) -> ()
          }
        }
        n146 = call "launch_test_1.vi"("Message Queues in"=w393, "test mode"=w388) -> ("error out"=w390:errorcluster, "Message Queues out"=w391:T8, "test mode out"=w392:T1)  [unwired: 7 in]
        n147 = call "launch_timer.vi"("error in (no error)"=w398, "Message Queues in"=w393, "test mode in"=w388) -> ("error out"=w399:errorcluster)  [unwired: 6 in, 2 out]
        n148 = call-poly "Enqueue Message.vi"("Message Array"=string[] ["Disable Start Button", "Idle"], "Message Queue"=w400) -> ("error out"=w402:errorcluster)  [unwired: 8 in, 1 out]
        n149 = call "turn_off_indicators.vi"("error in (no error)"=w390, "Message Queues in"=w391, "test mode in"=w392) -> ("error out"=w389:errorcluster)  [unwired: 6 in, 2 out]
        n150 = Merge Errors(w403, w389, w399, w402) -> (w405:errorcluster)
      }
      frame "Launch Test 2" {
        # "Something - Replace this message with functionality for your own application."
        n151 = Unbundle By Name(w413) -> ("test mode"=w412:T1)
        n152 = call "launch_test_2.vi"("Message Queues in"=w408, "test mode"=w412) -> ("error out"=w409:errorcluster)  [unwired: 9 in]
        n153 = call-poly "Enqueue Message.vi"("error in (no error)"=w416, "Message"="Idle", "Message Queue"=w411) -> ("error out"=w415:errorcluster)  [unwired: 7 in, 1 out]
        n154 = Merge Errors(w415, w409) -> (w417:errorcluster)
      }
      frame "Stop All Test" {
        n155 = flat-sequence {
          tunnel: errorcluster {"status"=FALSE, "code"=0, "source"=""} ("error constant") -> [w430]
          tunnel: [w430] -> w419
          frame #0 {
            n156 = local write "stp tmr"(TRUE ("stp tmr")) -> ()
          }
        }
        n157 = Unbundle By Name(w421) -> ("test mode"=w423:T1)
        n158 = call "launch_timer.vi"("error in (no error)"=w419, "Message Queues in"=w426, "test mode in"=w423) -> ("error out"=w424:errorcluster, "Message Queues out"=w425:T8, "test mode out"=w422:T1)  [unwired: 6 in]
        n159 = call "stop_all_test.vi"("error in (no error)"=w424, "Message Queues in"=w425, "test mode in"=w422) -> ("error out"=w418:errorcluster)  [unwired: 6 in, 2 out]
        n160 = Merge Errors(w429, w418) -> (w428:errorcluster)
      }
      frame "Enable Start Button" {
        n161 = Unbundle By Name(w435) -> ("Start Btn Refnum"=w434:refnum<vi>)
        n162 = property class="Bool"(reference=w434, "DisabledEnum"=T9."Enabled" ("Disabled")) -> (error out=w432:errorcluster)  [unwired: 1 in, 1 out]
        n163 = Merge Errors(w438, w432) -> (w436:errorcluster)
      }
      frame "Update Display" {
        # "#CodeRecommended - If you wish to decouple the Message Handling Loop from your user interface, consider creating User Events (like the \"Stop\" event in this VI) to message the Event Handling Loop whenever the user interface needs updating."
        # "Update Display - Convert the message data to a string to display in the Data Display indicator."
        n164 = Variant To Data(error in=w444, type="", Variant=w443) -> (data=→"Display":string, error out=w441:errorcluster)
        n165 = Merge Errors(w441) -> (w445:errorcluster)
      }
      frame "Error" {
        # "#CodeRecommended - If you ever change the name of this \"Error\" message, you'll need to update the name in the Check Loop Error.vi as well."
        # "#CodeRecommended - Consider creating a system for logging errors in some way. These errors are for notification purposes only. Handling of specific errors should be performed in the message frames that generated the error."
        # "Error - Display an error dialog. This message is sent by the \"Error Handler\" VIs \nat the end of other loops in this application."
        n166 = Variant To Data(error in=w454, type=errorcluster {"status"=FALSE, "code"=0, "source"=""} ("error constant"), Variant=w452) -> (data=w447:errorcluster, error out=w450:errorcluster)
        n167 = call "error_messages.vi"("error in (no error)"=w447) -> ()  [unwired: 10 in, 1 out]
        n168 = Merge Errors(w450) -> (w449:errorcluster)
      }
      frame "Confirm Quit" {
        # "#CodeNeeded - If you want to provide an \"Are you sure\" dialog (or some other notification) before the application exits, place that code here. This message is typically sent from a Panel Close? event."
        # "Confirm Quit - Message that can confirm whether or not the user wants to exit the application."
        n169 = Variant To Data(type="", Variant=w459) -> (data=w458:string, error out=w457:errorcluster)  [unwired: 1 in]
        n170 = Two Button Dialog(message=w458, 2:"Yes" ("T button name (\"OK\")")) -> (T button?=w462:bool)  [unwired: 1 in]
        n171 = case shown="True" w462 {
          tunnel: [string[] ["Idle"] string[] ["Exit", "Turn Off Indicators"]] -> w456
          frame False {
          }
          frame True {
          }
        }
        n172 = call-poly "Enqueue Message.vi"("Priority Message? Array"=bool[] [TRUE, TRUE], "error in (no error)"=w468, "Message Array"=w456, "Message Queue"=w464) -> ("error out"=w465:errorcluster)  [unwired: 6 in, 1 out]
        n173 = Merge Errors(w465, w457) -> (w466:errorcluster)
      }
      frame "Turn Off Indicators" {
        w472 = ""
        n174 = Bundle By Name(cluster=w474, "Delay Time"=0.0, "prms"=T10 {"1st tst"=0.0, "2nd tst"=0.0, "overlap"=0.0, "tst time"=0.0, "delay"=0.0}) -> (w473:T5)
        n175 = local write "GB ID"(w472) -> ()
        n176 = local write "I/F type"(w472) -> ()
        n177 = local write "HP ID"(w472) -> ()
      }
      frame "Exit" {
        # "Stop the VI"
        # "Release the message queue reference"
        # "Exit - Exit the application."
        n178 = Variant To Data(type=errorcluster {"status"=FALSE, "code"=0, "source"=""} ("error constant"), Variant=w485) -> (data=w481:errorcluster)  [unwired: 1 in, 1 out]
        n179 = call "error_messages.vi"("error in (no error)"=w481) -> ()  [unwired: 10 in, 1 out]
        n180 = Unbundle By Name(w479) -> ("test mode"=w478:T1)
        n181 = Release Queue(queue=w491, error in (no error)=w487) -> (error out=w484:errorcluster)  [unwired: 1 in, 2 out]
        n182 = call "exit_tasks.vi"("Message Queues out"=w480, "test mode"=w478) -> ("error out"=w482:errorcluster)  [unwired: 9 in]
        n183 = call "Fire User Event - Stop.vi"("User Event - Stop"=w488) -> ("error out"=w483:errorcluster)  [unwired: 10 in]
        n184 = Merge Errors(w484, w483, w482) -> (w489:errorcluster)
      }
      frame "---Copy This Frame---" {
        # "Duplicate this frame when creating new messages. Change this comment in the duplicated frame to describe this message."
        n185 = Merge Errors(w496) -> (w494:errorcluster)
      }
    }
    n186 = Unbundle By Name(w301) -> ("test mode"=→"tst mod":T1, "prms.delay"=→"delay":dbl, "prms.1st tst"=→"1st tst":dbl, "prms.2nd tst"=→"2d tst":dbl, "prms.overlap"=→"overlap":dbl, "prms.tst time"=→"tst time":dbl)
    n187 = call "Error Handler - Message Handling Loop_for_MAIN_loop.vi"("error in (no error)"=w313, "Message Queue"=w292) -> ("dup error in"=w307:errorcluster)  [unwired: 8 in, 1 out]
  }
  n188 = while {
    shift-right: [w507] -> _
    shift-left: T3 {"Status GB"="", "Results GB"="", "GB Pass/Fail"={"PASS"=FALSE, "FAIL"=FALSE}} ("GB Data") -> [w514]
    tunnel: w35 -> [w513]
    tunnel: [w502] -> w15
    tunnel: w6 -> [w509]
    tunnel: w5 -> [w499]
    stop <- w510 stop-if-true
    # "GB TEST LOOP"
    # "Message Handling Loop"
    n189 = Unbundle By Name(w499) -> ("GB Test"=w506:refnum<queue>)
    n190 = Unbundle By Name(w509) -> ("test mode"=w498:T1, "Rsrc name for 19572"=w508:refnum<visa-resource-name>)
    n191 = call "Dequeue Message.vi"("error in (no error)"=w513, "Message Queue"=w506) -> ("error out"=w512:errorcluster, "Message Data"=w511:variant, "Message"=w501:string, "dup Message Queue"=w497:refnum<queue>)  [unwired: 6 in]
    n192 = case "Message Cases" shown="\"Initialize\"" w501 {
      selector: w501 -> [w515 _ _ _ _ _ _ _ _ _ _ _ _ _]
      tunnel: w497 -> [_ _ _ _ _ w553 _ _ _ w594 _ _ w622 _]
      tunnel: w512 -> [_ w527 w531 w536 w541 w555 w572 w586 w588 w593 w599 w608 w618 w625]
      tunnel: [w516 w526 w531 w536 w540 w556 w571 w583 w590 w592 w600 w602 w619 w623] -> w503
      tunnel: w514 -> [w517 w529 w530 w535 w537 w551 w569 w585 w591 w595 w601 w607 w613 w624]
      tunnel: [w517 w529 w530 w534 w537 w550 w568 w585 w591 w595 w601 w607 w612 w624] -> w507
      tunnel: [_ _ _ _ _ _ _ _ _ _ _ _ TRUE _] -> w510
      tunnel: w511 -> [_ _ _ _ _ _ _ _ _ _ w598 w606 w616 _]
      tunnel: w508 -> [_ _ _ _ w542 w552 w570 _ w589 _ _ _ _ _]
      tunnel: w499 -> [_ _ _ _ _ _ w566 _ _ _ _ _ _ _]
      tunnel: w498 -> [_ _ _ _ _ _ w573 _ _ _ _ _ _ _]
      frame Default {
        # "'Default' case only runs if there is a message that isn't defined in any of the other cases. \nOutput a programming error."
        n193 = xnode "Error Ring"("parameter 0"=w515) -> ("error out"=w516:errorcluster)
      }
      frame "Initialize" {
        w528 = 0.0
        n194 = local write "GB test"(w528) -> ()
        n195 = property on="GB test" class="Slide (strict)"("Scale.Maximum"=w528, "Scale.Minimum"=w528) -> (error out=w525:errorcluster)  [unwired: 2 in, 1 out]
        n196 = Merge Errors(w527, w525) -> (w526:errorcluster)
      }
      frame "Idle" {
      }
      frame "Turn Off Status Inds" {
        w533 = ""
        n197 = Bundle By Name(cluster=w535, "Status GB"=w533, "Results GB"=w533, "GB Pass/Fail"=cluster{"PASS":bool, "FAIL":bool} {"PASS"=FALSE, "FAIL"=FALSE}) -> (w534:T3)
      }
      frame "Start GB Test" {
        n198 = call "19572 Series START.vi"("VISA resource in"=w542) -> ("error out"=w539:errorcluster)  [unwired: 9 in, 1 out]
        n199 = Merge Errors(w541, w539) -> (w540:errorcluster)
        n200 = call "stop_watch_w_feedback_node1.vi"("Command"=enum16{"Elapsed Time", "Reset"}."Reset") -> ()  [unwired: 10 in, 1 out]
      }
      frame "Check GB Results" {
        n201 = call "19572_Get_STATUS.vi"("VISA resource in"=w552) -> ("error out"=w546:errorcluster, "Status"=w545:string)  [unwired: 8 in, 1 out]
        n202 = Equal?(x=w545, y="RUNNING") -> (x = y?=w548:bool)
        n203 = Bundle By Name(cluster=w551, "Status GB"=w545) -> (w550:T3)
        n204 = case shown="False" w548 {
          tunnel: [string[] ["Read GB Results", "Enable Start Button"] string[] ["Check GB Results"]] -> w547
          frame False {
          }
          frame True {
          }
        }
        n205 = call "stop_watch_w_feedback_node1.vi"("Command"=enum16{"Elapsed Time", "Reset"}."Elapsed Time") -> ("Elapsed Time"=→"GB test":dbl)  [unwired: 10 in]
        n206 = call-poly "Enqueue Message.vi"("error in (no error)"=w555, "Message Array"=w547, "Message Queue"=w553) -> ("error out"=w554:errorcluster)  [unwired: 7 in, 1 out]
        n207 = Merge Errors(w554, w546) -> (w556:errorcluster)
      }
      frame "Read GB Results" {
        n208 = call "19572_pass_fail_parser.vi"("VISA resource in"=w570) -> ("error out"=w563:errorcluster, "Pass/Fail"=w565:cluster{"PASS":bool, "FAIL":bool}, "Code Results"=w567:string)  [unwired: 7 in, 1 out]
        n209 = Bundle By Name(cluster=w569, "Results GB"=w567, "GB Pass/Fail"=w565) -> (w568:T3)
        n210 = call "stop_hp_test_if_gb_test_fail.vi"("Message Queues in"=w566, "Pass/Fail"=w565) -> ("error out"=w564:errorcluster, "Message Queues out"=w560:T8, "Fail?"=w559:bool)  [unwired: 7 in]
        n211 = case shown="True" w559 {
          tunnel: [w574 w578] -> w562
          tunnel: errorcluster {"status"=FALSE, "code"=0, "source"=""} ("error constant") -> [w574 w577]
          tunnel: w573 -> [_ w576]
          tunnel: w560 -> [_ w575]
          frame False {
          }
          frame True {
            n212 = flat-sequence {
              tunnel: w577 -> [w580]
              tunnel: [w580] -> w579
              frame #0 {
                n213 = local write "stp tmr"(TRUE ("stp tmr")) -> ()
              }
            }
            n214 = call "launch_timer.vi"("error in (no error)"=w579, "Message Queues in"=w575, "test mode in"=w576) -> ("error out"=w578:errorcluster)  [unwired: 6 in, 2 out]
          }
        }
        n215 = Merge Errors(w572, w562, w564, w563) -> (w571:errorcluster)
      }
      frame "Enable Start Button" {
        n216 = property on="Start test" class="Bool"("DisabledEnum"=T9."Enabled" ("Disabled")) -> (error out=w582:errorcluster)  [unwired: 2 in, 1 out]
        n217 = Merge Errors(w586, w582) -> (w583:errorcluster)
      }
      frame "Stop GB Test" {
        n218 = call "19572 Series STOP.vi"("VISA resource in"=w589) -> ("error out"=w587:errorcluster)  [unwired: 9 in, 1 out]
        n219 = Merge Errors(w588, w587) -> (w590:errorcluster)
      }
      frame "Flush Queue" {
        n220 = Flush Queue(queue=w594, error in (no error)=w593) -> (error out=w592:errorcluster)  [unwired: 2 out]
      }
      frame "Update GB Display" {
        # "#CodeRecommended - If you wish to decouple the Message Handling Loop from your user interface, consider creating User Events (like the \"Stop\" event in this VI) to message the Event Handling Loop whenever the user interface needs updating."
        # "Update Display - Convert the message data to a string to display in the Data Display indicator."
        n221 = Variant To Data(error in=w599, type="", Variant=w598) -> (error out=w596:errorcluster)  [unwired: 1 out]
        n222 = Merge Errors(w596) -> (w600:errorcluster)
      }
      frame "Error" {
        # "#CodeRecommended - If you ever change the name of this \"Error\" message, you'll need to update the name in the Check Loop Error.vi as well."
        # "#CodeRecommended - Consider creating a system for logging errors in some way. These errors are for notification purposes only. Handling of specific errors should be performed in the message frames that generated the error."
        # "Error - Display an error dialog. This message is sent by the \"Error Handler\" VIs \nat the end of other loops in this application."
        n223 = Variant To Data(error in=w608, type=errorcluster {"status"=FALSE, "code"=0, "source"=""} ("error constant"), Variant=w606) -> (data=w604:errorcluster, error out=w603:errorcluster)
        n224 = call <vilib>:"Simple Error Handler.vi"("error in (no error)"=w604) -> ()  [unwired: 4 in, 5 out]
        n225 = Merge Errors(w603) -> (w602:errorcluster)
      }
      frame "Exit" {
        w611 = ""
        w615 = 0.0 ("HP test")
        # "Stop the VI"
        # "Release the message queue reference"
        # "#CodeNeeded - Add any required cleanup code here. Note that if 'Exit' was called as a result of an error, an error dialog will be displayed. Add any custom error handling for an 'Exit' condition here as well."
        # "Exit - Exit the application."
        n226 = Variant To Data(type=errorcluster {"status"=FALSE, "code"=0, "source"=""} ("error constant"), Variant=w616) -> (data=w610:errorcluster)  [unwired: 1 in, 1 out]
        n227 = call "error_messages.vi"("error in (no error)"=w610) -> ()  [unwired: 10 in, 1 out]
        n228 = Release Queue(queue=w622, error in (no error)=w618) -> (error out=w620:errorcluster)  [unwired: 1 in, 2 out]
        n229 = property on="GB test" class="Slide (strict)"("Scale.Maximum"=w615, "Scale.Minimum"=w615) -> (error out=w614:errorcluster)  [unwired: 2 in, 1 out]
        n230 = local write "GB test"(w615) -> ()
        n231 = Bundle By Name(cluster=w613, "Status GB"=w611, "Results GB"=w611, "GB Pass/Fail"=cluster{"PASS":bool, "FAIL":bool} {"PASS"=FALSE, "FAIL"=FALSE}) -> (w612:T3)
        n232 = Merge Errors(w620, w614) -> (w619:errorcluster)
      }
      frame "---Copy This Frame---" {
        # "Duplicate this frame when creating new messages.\nChange this comment in the duplicated frame to describe this message."
        n233 = Merge Errors(w625) -> (w623:errorcluster)
      }
    }
    n234 = Unbundle By Name(w507) -> ("Status GB"=→"GB tst st":string, "Results GB"=→"GB tst reslts":string, "GB Pass/Fail"=→"GB Pass/Fail":cluster{"PASS":bool, "FAIL":bool})
    n235 = call "Error Handler - Message Handling Loop_for_GB_loop.vi"("error in (no error)"=w503, "Message Queue"=w497) -> ("dup error in"=w502:errorcluster)  [unwired: 8 in, 1 out]
  }
  n236 = Unregister For Events(event registration refnum=w27, error in=w26) -> (error out=w28:errorcluster)
  n237 = Merge Errors(w23, w28, w15, w24, w7) -> (w21:errorcluster)
  n238 = call "close_visa_resources.vi"("error in (no error)"=w21, "VISA in"=w22) -> ("error out"=w1:errorcluster)  [unwired: 9 in]
  n239 = Destroy User Event(user event=w34, error in=w1) -> (error out=w3:errorcluster)
  n240 = call "Destroy User Event - Stop.vi"("error in (no error)"=w3, "User Event - Stop"=w29) -> ("error out"=w20:errorcluster)  [unwired: 9 in]
  n241 = disable-structure shown="RUN_TIME_ENGINE==True" {
    disable-tunnel: w20 -> [_ _]
    frame condition #0 (active) {
    }
    frame condition #1 {
      # "Call Quit LabVIEW if running as a built application."
      n242 = Quit LabVIEW() -> ()  [unwired: 1 in]
    }
  }
